vi "programa 6.vi"() -> ()   [LabVIEW 2011]
panel:
  out "Alarma":bool
  out "Temperatura":i32(slide) scale=0.0..100.0
  out "Cuarta":bool
  out "Segunda":bool
  out "Tercera":bool
  out "Primera":bool
  out "Velocidad":i32(knob) scale=0.0..180.0
  # "Debera de generar la velocidad en numero entero.\nLuego de acuerdo a la siguiente tabla:\n\n1-30 primera\n31-50 segunda\n51-85 tercera\n86-180 cuarta\n\nDebera de encender las luces de los cambios.\n\nEncender la alamarma cuando la temperatura sobrepase\nlos 80 grados y la velocidad es mayor a 150."
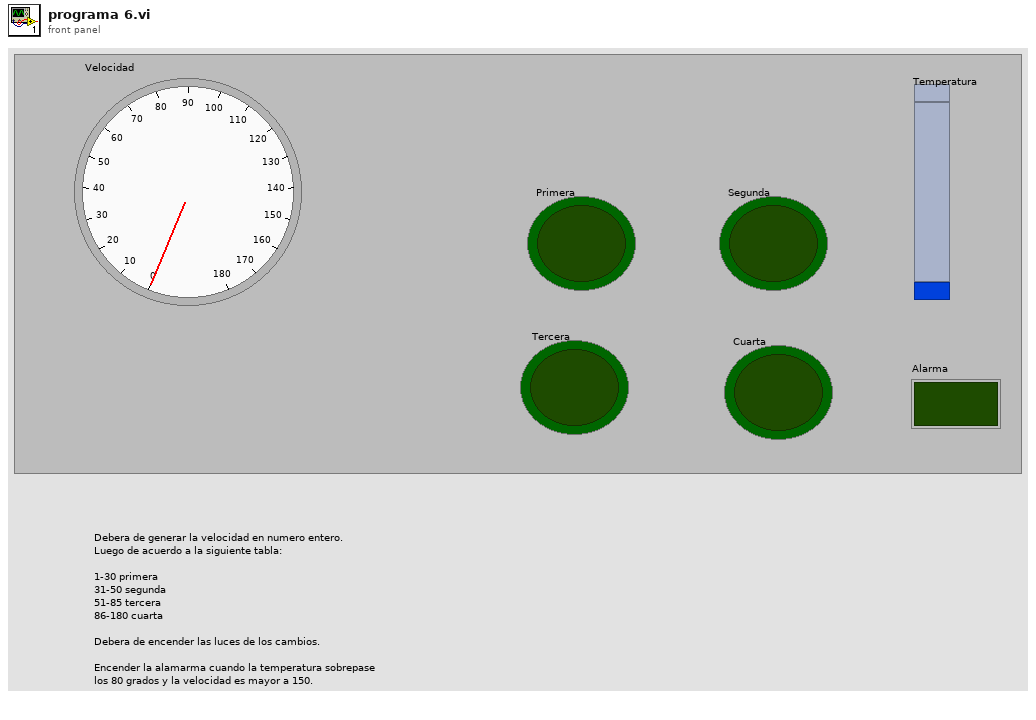
[diagram p1: front panel]
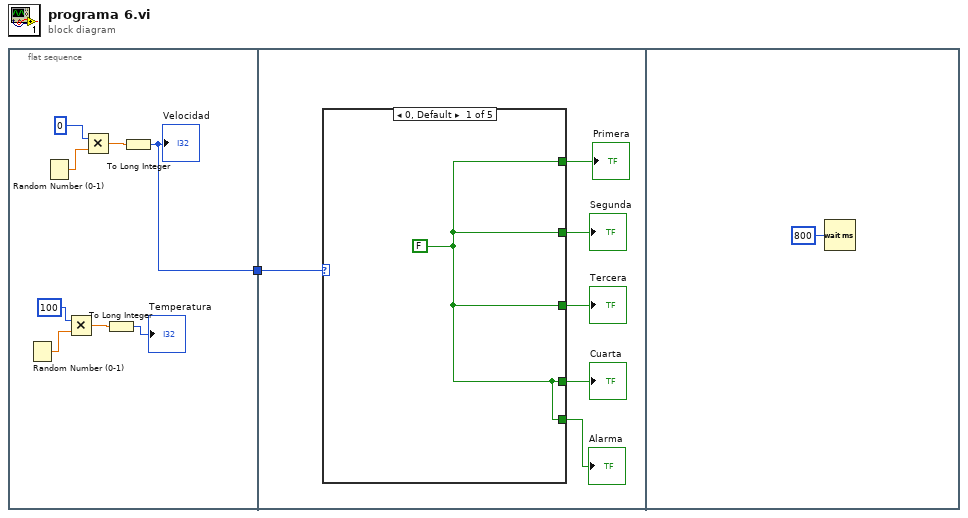
[diagram p0: block diagram]
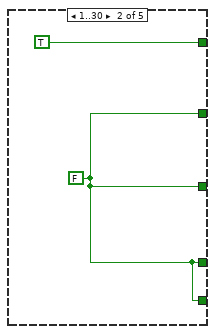
[diagram p2: hidden frame]
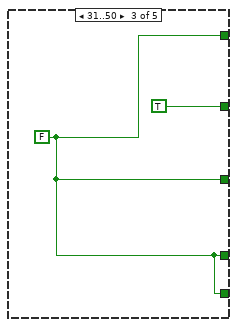
[diagram p3: hidden frame]
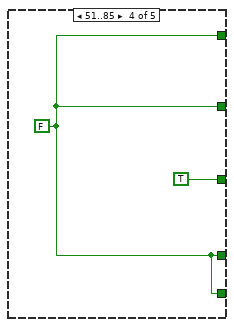
[diagram p4: hidden frame]
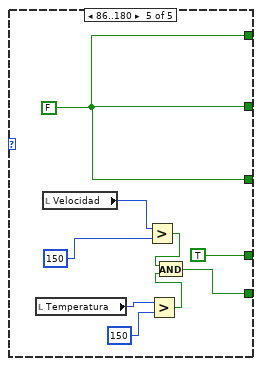
[diagram p5: hidden frame]
diagram:
  n1 = flat-sequence {
    tunnel: [w6] -> w1
    tunnel: w1 -> [w15]
    frame #0 {
      n2 = Random Number (0-1)() -> (number: 0 to 1=w5:dbl)
      n3 = Random Number (0-1)() -> (number: 0 to 1=w7:dbl)
      n4 = Multiply(x=100, y=w5) -> (x*y=w3:dbl)
      n5 = Multiply(x=0, y=w7) -> (x*y=w9:dbl)
      n6 = To Long Integer(number=w3) -> (32bit integer=→"Temperatura":i32)
      n7 = To Long Integer(number=w9) -> (32bit integer=w6:i32)
      "Velocidad" <- w6
    }
    frame #1 {
      n8 = case shown="0, Default" w15 {
        tunnel: [w16 TRUE w19 w21 w30] -> w14
        tunnel: [w16 w17 w19 w21 TRUE] -> w13
        tunnel: [w16 w17 w19 TRUE w30] -> w12
        tunnel: [w16 w17 TRUE w21 w30] -> w11
        tunnel: [w16 w17 w19 w21 w24] -> w10
        frame 0, Default {
          w16 = FALSE
        }
        frame 1..30 {
          w17 = FALSE
        }
        frame 31..50 {
          w19 = FALSE
        }
        frame 51..85 {
          w21 = FALSE
        }
        frame 86..180 {
          w30 = FALSE
          n9 = local read "Temperatura"() -> (w23:i32)
          n10 = local read "Velocidad"() -> (w29:i32)
          n11 = Greater?(x=w29, y=u32 150 ("milliseconds to wait")) -> (0:w26:bool)
          n12 = Greater?(x=w23, y=u32 150 ("milliseconds to wait")) -> (0:w25:bool)
          n13 = And(x=w26, y=w25) -> (x .and. y?=w24:bool)
        }
      }
      "Primera" <- w14
      "Segunda" <- w11
      "Tercera" <- w12
      "Cuarta" <- w13
      "Alarma" <- w10
    }
    frame #2 {
      n14 = Wait (ms)(milliseconds to wait=u32 800) -> ()  [unwired: 1 out]
    }
  }
